vi "ble_delete_repeated_scan_responses.vi"(11 "Scan Responses":string[][](array[string])) -> (3 "Unique Scan Responses":string[][](array[string]))   [LabVIEW 2015]
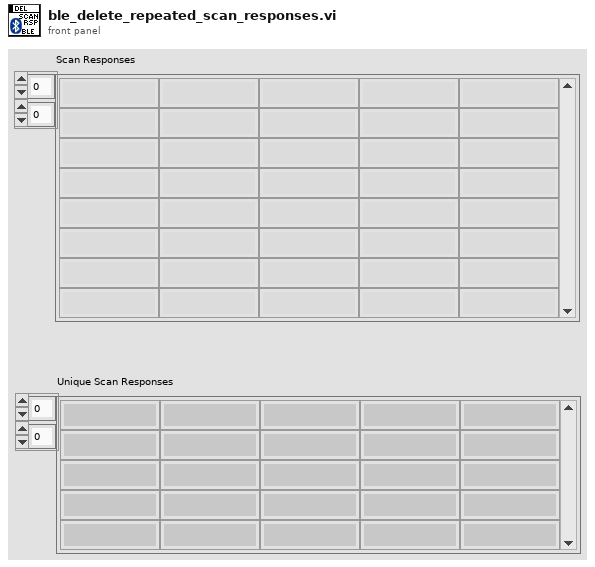
[diagram p1: front panel]
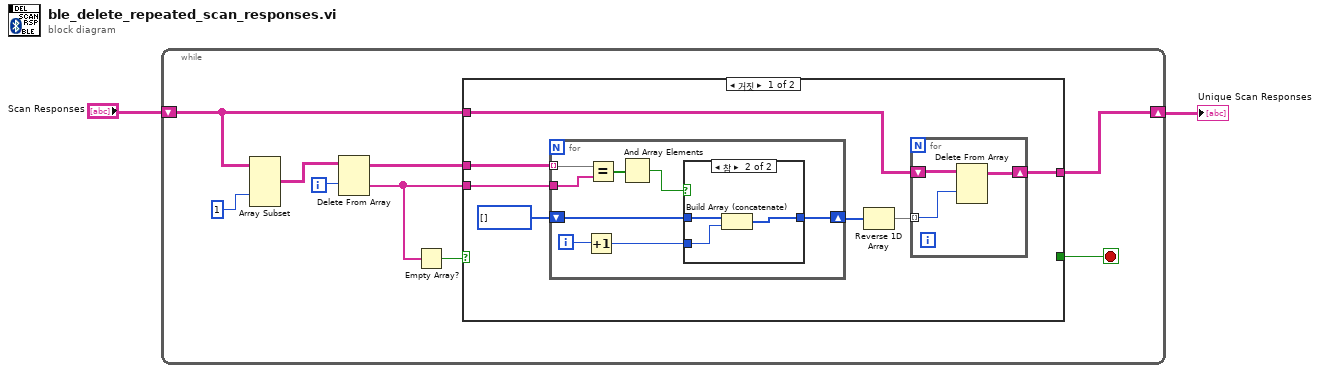
[diagram p0: block diagram]
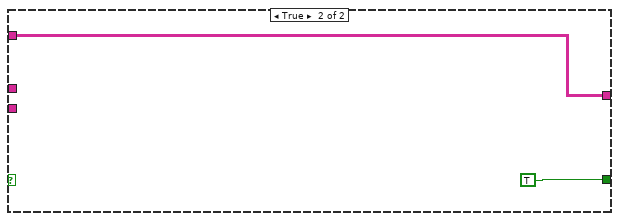
[diagram p3: hidden frame]
diagram:
  n1 = while {
    shift-right: [w6] -> w2
    shift-left: "Scan Responses" -> [w7]
    i -> [w11]
    stop <- w3 stop-if-true
    n2 = Array Subset(array=w7, index (col)=1 ("index")) -> (w9:string[][])  [unwired: 3 in]
    n3 = Delete From Array(array=w9, index (row)=w11) -> (deleted portion=w5:string[], array with subset deleted=w8:string[][])  [unwired: 2 in]
    n4 = Empty Array?(array=w5) -> (empty?=w4:bool)
    n5 = case shown="거짓" w4 {
      tunnel: w8 -> [w18 _]
      tunnel: w7 -> [w16 w35]
      tunnel: [w15 w35] -> w6
      tunnel: w5 -> [w12 _]
      tunnel: [_ TRUE] -> w3
      frame False {
        n6 = for {
          tunnel: w18 -> [w29] mode=indexing
          tunnel: w12 -> [w28]
          shift-right: [w22] -> w13
          shift-left: i32[] [] -> [w25]
          i -> [w27]
          n7 = Increment(x=w27) -> (x+1=w24:i32)
          n8 = Equal?(x=w29, y=w28) -> (x = y?=w26:bool[])
          n9 = And Array Elements(Boolean array=w26) -> (logical AND=w23:bool)
          n10 = case shown="참" w23 {
            tunnel: w25 -> [w30 w33]
            tunnel: w24 -> [_ w32]
            tunnel: [w30 w31] -> w22
            frame False {
            }
            frame True {
              n11 = Build Array (concatenate)(w33, w32) -> (w31:i32[])
            }
          }
        }
        n12 = Reverse 1D Array(array=w13) -> (reversed array=w14:i32[])
        n13 = for {
          shift-right: [w19] -> w15
          shift-left: w16 -> [w21]
          tunnel: w14 -> [w20] mode=indexing
          n14 = Delete From Array(array=w21, index (row)=w20) -> (array with subset deleted=w19:string[][])  [unwired: 2 in, 1 out]
        }
      }
      frame True {
      }
    }
  }
  "Unique Scan Responses" <- w2
